vi "Simulate DAQ Error.vi"(9 "Iteration":i32) -> (0 "Error?":bool, 1 "error out":errorcluster)   [LabVIEW 2011]
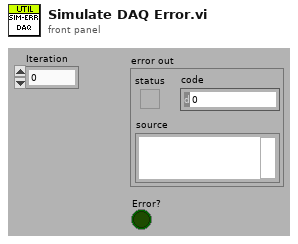
[diagram p1: front panel]
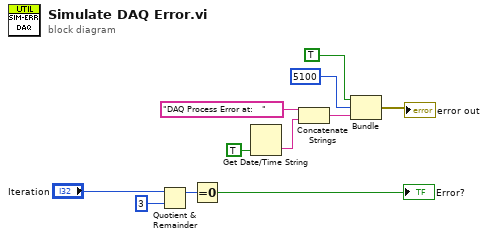
[diagram p0: block diagram]
diagram:
  n1 = Quotient & Remainder(x="Iteration", y=3) -> (x-y*floor(x/y)=w9:i32)  [unwired: 1 out]
  n2 = Equal To 0?(x=w9) -> (x = 0?=→"Error?":bool)
  n3 = Get Date/Time String(want seconds? (F)=TRUE) -> (time string=w10:string)  [unwired: 2 in, 1 out]
  n4 = Concatenate Strings("DAQ Process Error at:   ", w10) -> (w6:string)
  n5 = Bundle(TRUE, 5100, w6) -> (→"error out":errorcluster)  [unwired: 1 in]
